vi "Fill_empry_with_zero_for_year_duration.vi"(11 "duration In":string[](array[string])) -> (3 "duration out":string[](array[string]))   [LabVIEW 2017]
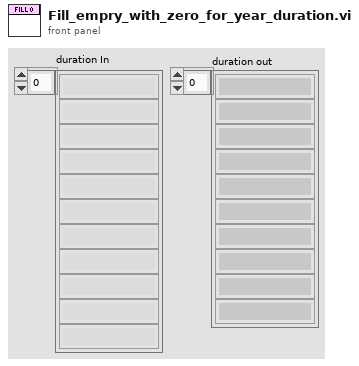
[diagram p1: front panel]
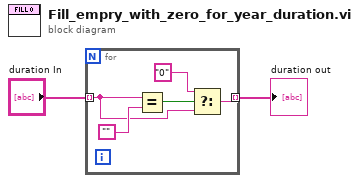
[diagram p0: block diagram]
diagram:
  n1 = for {
    tunnel: "duration In" -> [w5] mode=indexing
    tunnel: [w3] -> w2 mode=indexing
    n2 = Equal?(x=w5, y="") -> (x = y?=w6:bool)
    n3 = Select(t="0", s=w6, f=w5) -> (s? t:f=w3:string)
  }
  "duration out" <- w2
